vi "Log Event.vi"(0 "TDMS Log In":refnum<class "TDMS Logger.lvclass">, 5 "Group Name (Events)":string="Events", 7 "Channels Names":string[](array[string]), 9 "String Data":string[](array[string]), 11 "Error In":errorcluster) -> (4 "TDMS Log Out":refnum<class "TDMS Logger.lvclass">, 15 "Error Out":errorcluster)   [LabVIEW 2019, in "TDMS Logger.lvlib" / "TDMS Logger.lvclass"]
doc: "Log a 1D array of strings to the TDMS file. Each element corresponds to one event that you want to log to the file. Along with the events that you wire there will be added one Time column, informing about the time of the call of this function.\n\nProviding meaningful names as the channel names is required because they will describe the nature of the logged events."
uses:
  TDMS Logger.lvclass
  TDMS Logger.lvclass/TDMS Logger.ctl
  _Typedefs/Data Type.ctl
  _Typedefs/Log Message.ctl
  _Typedefs/Log Action.ctl
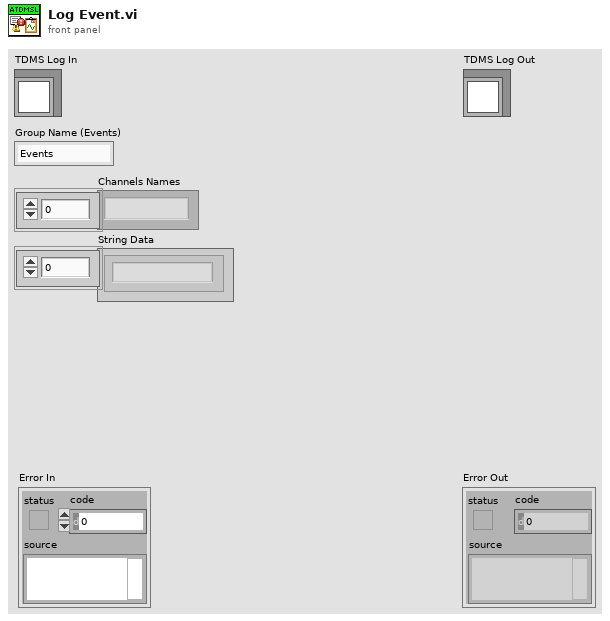
[diagram p1: front panel]
types:
  T1 = typedef "TDMS Logger.lvlib/TDMS Logger.lvclass/Data Type.ctl" = enum16{"I16", "I8", "String", "U16", "U8", "Waveform", "Double", "Single"}
  T2 = typedef "TDMS Logger.lvlib/TDMS Logger.lvclass/Log Message.ctl" = cluster{"Log Action":T3, "Variant":variant, "Data Type":T1, "Group Name":string, "Channels Names":string[]}
  T3 = typedef "TDMS Logger.lvlib/TDMS Logger.lvclass/Log Action.ctl" = enum16{"Handle Old Files", "Status Update", "Stop", "Log Data", "Initialize"}
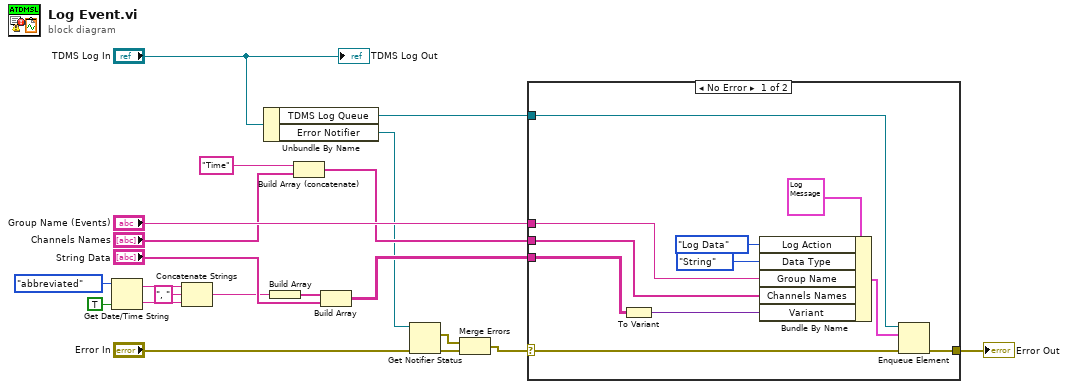
[diagram p0: block diagram]
diagram:
  n1 = Get Date/Time String(date format (0)=enum16{"short", "long", "abbreviated"}."abbreviated", want seconds? (F)=TRUE) -> (date string=w15:string, time string=w14:string)  [unwired: 1 in]
  n2 = Concatenate Strings(w15, ", " ("string"), w14) -> (w12:string)
  n3 = Unbundle By Name("TDMS Log In") -> ("TDMS Log Queue"=w2:refnum<queue>, "Error Notifier"=w8:refnum<notifier>)
  n4 = Build Array(w12) -> (w11:string[])
  n5 = Build Array (concatenate)("Time", "Channels Names") -> (w17:string[])
  n6 = Build Array(w11, "String Data") -> (w10:string[][])
  n7 = Get Notifier Status(notifier=w8, error in (no error)="Error In") -> (current notification=w5:errorcluster, error out=w6:errorcluster)  [unwired: 3 out]
  n8 = Merge Errors(w5, w6) -> (w4:errorcluster)
  n9 = case shown="No Error" w4 {
    selector: w4 -> [w25 w33]
    tunnel: [w24 w33] -> w21
    tunnel: "Group Name (Events)" -> [w27 _]
    tunnel: w17 -> [w26 _]
    tunnel: w10 -> [w23 _]
    tunnel: w2 -> [w28 _]
    frame No Error {
      n10 = To Variant(anything=w23) -> (Variant=w22:variant)
      n11 = Bundle By Name(cluster=T2 {"Log Action"=enum."Stop", "Variant"=variant, "Data Type"=enum."String", "Group Name"="", "Channels Names"=[]} ("element"), "Log Action"=Log_Action."Log Data", "Data Type"=Data_Type."String", "Group Name"=w27, "Channels Names"=w26, "Variant"=w22) -> (w31:T2)
      n12 = Enqueue Element(queue=w28, element=w31, error in (no error)=w25) -> (error out=w24:errorcluster)  [unwired: 1 in, 2 out]
    }
    frame Error {
    }
  }
  "Error Out" <- w21
  "TDMS Log Out" <- "TDMS Log In"
